vi "CH1.vi"() -> ()   [LabVIEW 2021]
panel:
  in  "CH1":cluster{"CH1 Array":dbl[], "CH1 Message":string}
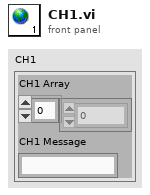
[diagram p1: front panel]
diagram:
